vi "Write LogicIO Obj.vi"(10 "Hardware.lvlib:LogicIO.lvlib:LogicIO.lvclass":refnum<class "LogicIO.lvclass">, 11 "LogicIO Configuration in":refnum<class "LogicIO Configuration.lvclass">) -> (3 "LogicIO Configuration out":refnum<class "LogicIO Configuration.lvclass">)   [LabVIEW 2016, in "Hardware.lvlib" / "LogicIO.lvlib" / "LogicIO Configuration.lvclass"]
uses:
  <userlib>/Common Components/Hardware/LogicIO/LogicIO Config/LogicIO Configuration.lvclass
  <userlib>/Common Components/Hardware/LogicIO/LogicIO/LogicIO.lvclass
  <userlib>/Common Components/Hardware/LogicIO/LogicIO Config/LogicIO Configuration.lvclass/LogicIO Configuration.ctl
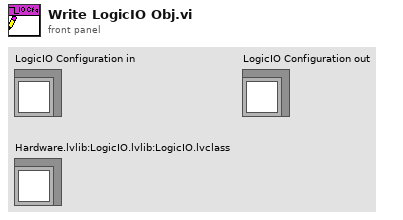
[diagram p1: front panel]
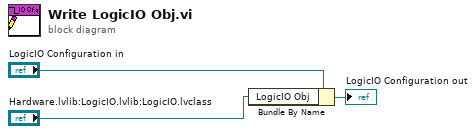
[diagram p0: block diagram]
diagram:
  n1 = Bundle By Name(cluster="LogicIO Configuration in", "LogicIO Obj"="Hardware.lvlib:LogicIO.lvlib:LogicIO.lvclass") -> (→"LogicIO Configuration out":refnum<class "LogicIO Configuration.lvclass">)
